vi "test Loopback_Acyclic Messages.vi"(8 "error in":errorcluster, 11 "TestCase in":refnum<class "Single Core Acyclic Loopback.lvclass">) -> (0 "error out":errorcluster, 3 "TestCase out":refnum<class "Single Core Acyclic Loopback.lvclass">)   [LabVIEW 2020, in "Single Core Acyclic Loopback.lvclass"]
uses:
  Single Core Acyclic Loopback.lvclass
  C:/Git/niveristand-custom-device-testing-tools/VeriStandTestCase/VeriStandTestCase.lvclass
  <vilib>/numeric/Random Number (Range) I64.vi
  <vilib>/numeric/sub_Random U32.vi
  <vilib>/NI VeriStand/Execution/Workspace/NI VeriStand - Set Multiple Channel Values.vi
  <vilib>/addons/_JKI Toolkits/VI Tester/TestCase.llb/TestCase.lvclass
  <vilib>/NI VeriStand/Execution/Workspace/NI_VS Workspace ExecutionAPI.lvlib
  niveristand-custom-device-testing-tools/VeriStandTestUtilities/VeriStandTestUtilities.lvlib
  C:/Program Files (x86)/National Instruments/LabVIEW 2020/vi.lib/addons/_JKI Toolkits/VI Tester/TestCase.llb/TestCase.lvclass
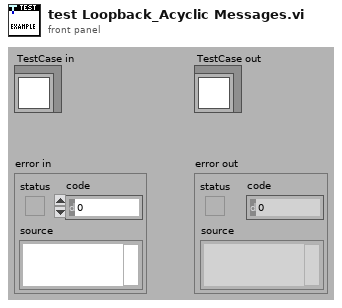
[diagram p1: front panel]
types:
  T1 = typedef "NI_VS Workspace ExecutionAPI.lvlib/WorkspaceAPI.ctl" = refnum<k24>
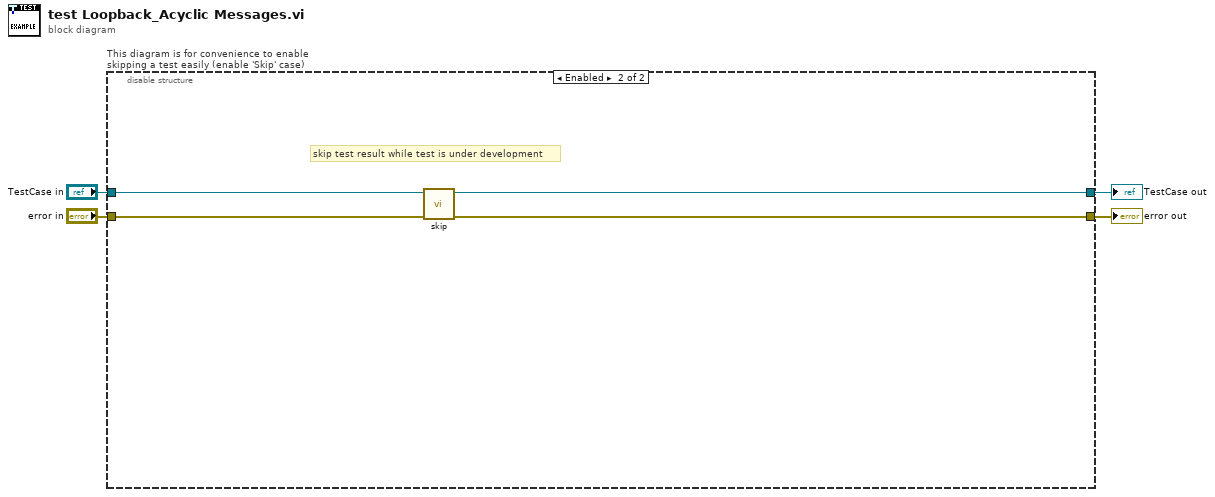
[diagram p0: block diagram]
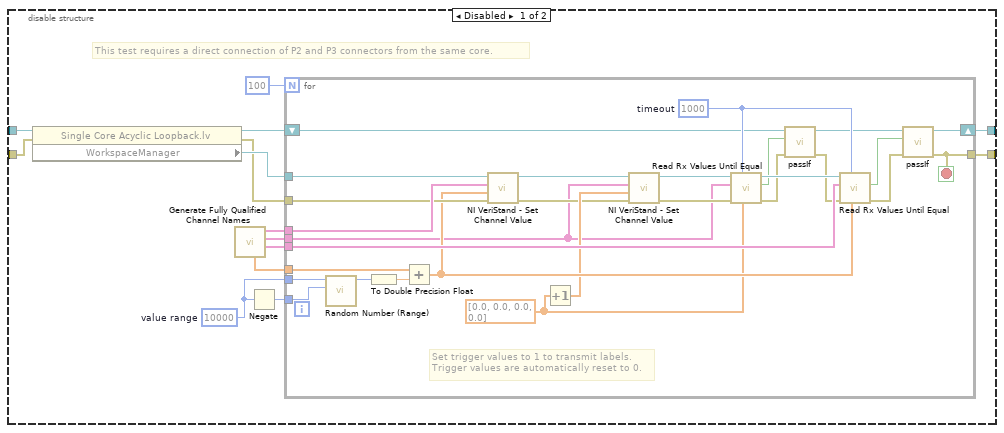
[diagram p2: hidden frame]
diagram:
  n1 = disable-structure "This diagram is for convenience to enable skipping a test easily (enable 'Skip' case)" shown="Enabled" {
    disable-tunnel: "TestCase in" -> [w18 w50]
    disable-tunnel: [w6 w48] -> w1
    disable-tunnel: [w5 w49] -> w3
    disable-tunnel: "error in" -> [w17 w47]
    frame Disabled {
      w15 = i64 10000  # value range
      # "This test requires a direct connection of P2 and P3 connectors from the same core."
      n2 = property class="Single Core Acyclic Loopback.lv"(reference=w18, error in=w17) -> (reference out=w9:refnum<class "Single Core Acyclic Loopback.lvclass">, error out=w11:errorcluster, "WorkspaceManager"=w12:T1)
      n3 = call "Generate Fully Qualified Channel Names.vi"() -> ("Rx channels"=w10:string[], "trigger channels"=w7:string[], "Tx channels"=w13:string[], "channel index"=w16:dbl[])  [unwired: 8 in]
      n4 = Negate(x=w15) -> (-x=w14:i64)
      n5 = for {
        N: 100 -> [_]
        tunnel: w16 -> [w44]
        tunnel: w15 -> [w43]
        tunnel: w14 -> [w42]
        tunnel: w13 -> [w41]
        tunnel: w12 -> [w40]
        tunnel: w11 -> [w39]
        tunnel: w10 -> [w38]
        shift-right: [w36] -> w6
        shift-left: w9 -> [w20]
        tunnel: [w34] -> w5
        tunnel: w7 -> [w26]
        stop <- w34 stop-if-true
        w25 = dbl[] [0.0, 0.0, 0.0, 0.0]
        w24 = 1000  # timeout
        # "Set trigger values to 1 to transmit labels. \nTrigger values are automatically reset to 0."
        n6 = call-poly <vilib>:"Random Number (Range).vi"("lower bound (-100)"=w42, "upper bound (100)"=w43) -> ("number"=w46:i64)  [unwired: 9 in]
        n7 = To Double Precision Float(number=w46) -> (double precision float=w45:dbl)
        n8 = Add(x=w44, y=w45) -> (x+y=w35:dbl[])
        n9 = call-poly <vilib>:"NI VeriStand - Set Channel Value.vi"("error in (no error)"=w39, "Values"=w35, "Channels"=w41, "WorkspaceManager in"=w40) -> ("error out"=w30:errorcluster, "WorkspaceManager out"=w31:T1)  [unwired: 6 in]
        n10 = Increment(x=w25) -> (x+1=w32:dbl[])
        n11 = call-poly <vilib>:"NI VeriStand - Set Channel Value.vi"("error in (no error)"=w30, "Values"=w32, "Channels"=w26, "WorkspaceManager in"=w31) -> ("error out"=w28:errorcluster, "WorkspaceManager out"=w29:T1)  [unwired: 6 in]
        n12 = call "Read Rx Values Until Equal.vi"("expected values"=w25, "timeout (1000 ms)"=w24, "error in"=w28, "Rx aliases"=w26, "workspace manager in"=w29) -> ("error out"=w21:errorcluster, "values equal expected"=w19:bool, "workspace manager out"=w27:T1)  [unwired: 4 in]
        n13 = call-dynamic "passIf.vi"("error in (no error)"=w21, "pass"=w19, "TestCase in"=w20) -> ("error out"=w22:errorcluster, "TestCase out"=w23:refnum<class "Single Core Acyclic Loopback.lvclass">)  [unwired: 7 in]
        n14 = call "Read Rx Values Until Equal.vi"("expected values"=w35, "timeout (1000 ms)"=w24, "error in"=w22, "Rx aliases"=w38, "workspace manager in"=w27) -> ("error out"=w37:errorcluster, "values equal expected"=w33:bool)  [unwired: 4 in, 1 out]
        n15 = call-dynamic "passIf.vi"("error in (no error)"=w37, "pass"=w33, "TestCase in"=w23) -> ("error out"=w34:errorcluster, "TestCase out"=w36:refnum<class "Single Core Acyclic Loopback.lvclass">)  [unwired: 7 in]
      }
    }
    frame Enabled {
      # "skip test result while test is under development"
      n16 = call <vilib>:"skip.vi"("error in (no error)"=w47, "TestCase in"=w50) -> ("error out"=w49:errorcluster, "TestCase out"=w48:refnum<class "Single Core Acyclic Loopback.lvclass">)  [unwired: 8 in]
    }
  }
  "error out" <- w3
  "TestCase out" <- w1
